vi "Send Commands.vi"(4 "message attributes":T1[](array[typedef]), 6 "timeout (-1 ms)":i32=-1, 8 "error in (no error)":errorcluster, 9 "message values":string[](array[string]), 10 "message names":string[](array[string]), 11 "VeriStand Comm in":refnum<class "VeriStand Comm.lvclass">) -> (0 "error out":errorcluster, 3 "VeriStand Comm out":refnum<class "VeriStand Comm.lvclass">)   [LabVIEW 2020, in "NI VeriStand Addon Network Comm.lvlib" / "VeriStand Comm.lvclass"]
uses:
  VeriStand Comm.lvclass
  VeriStand Comm.lvclass/VeriStand Comm.ctl
  <vilib>/NI/AMC/AMC.lvlib
  <vilib>/NI/Tools/Keyed Array/KeyedArray.ctl
  <vilib>/NI/Tools/Keyed Array/Tools_KeyedArray.lvlib
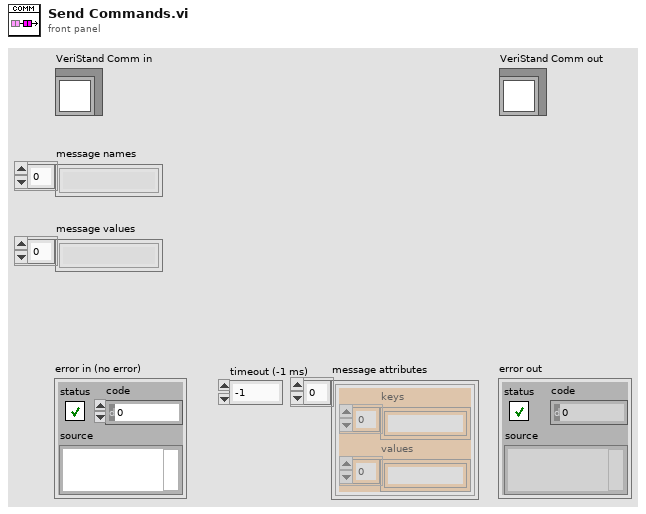
[diagram p1: front panel]
types:
  T1 = typedef "Tools_KeyedArray.lvlib/KeyedArray.ctl" = cluster{"keys":string[], "values":string[]}
  T2 = typedef "AMC.lvlib/Message Queue.ctl" = refnum<queue>
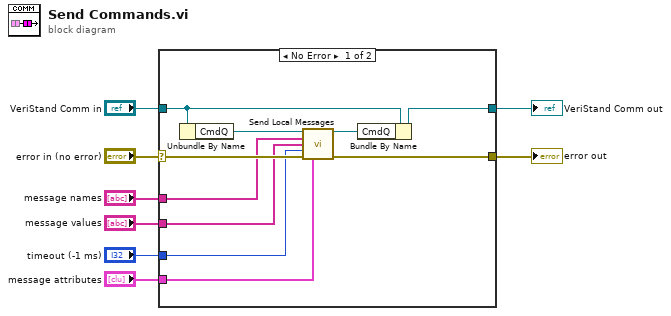
[diagram p0: block diagram]
diagram:
  n1 = case shown="No Error" "error in (no error)" {
    selector: "error in (no error)" -> [w17 w20]
    tunnel: [w18 w20] -> w7
    tunnel: [w12 w19] -> w5
    tunnel: "VeriStand Comm in" -> [w13 w19]
    tunnel: "message values" -> [w10 _]
    tunnel: "timeout (-1 ms)" -> [w16 _]
    tunnel: "message names" -> [w11 _]
    tunnel: "message attributes" -> [w9 _]
    frame No Error {
      n2 = Unbundle By Name(w13) -> ("CmdQ"=w15:T2)
      n3 = call <vilib>:"Send Local Messages.vi"("message queue in"=w15, "message names"=w11, "message values"=w10, "timeout (-1 ms)"=w16, "error in"=w17, "message attributes"=w9) -> ("message queue out"=w14:T2, "error out"=w18:errorcluster)  [unwired: 7 in, 1 out]
      n4 = Bundle By Name(cluster=w13, "CmdQ"=w14) -> (w12:refnum<class "VeriStand Comm.lvclass">)
    }
    frame Error {
    }
  }
  "error out" <- w7
  "VeriStand Comm out" <- w5
